vi "SCM Host Calibration.vi"() -> ()   [LabVIEW 2015]
uses:
  <vilib>/addons/Software Calibration Management/XControls/TBL2D.xctl
  <vilib>/addons/Software Calibration Management/XControls/TBL1D.xctl
panel:
  in  "stop":bool
  in  "Calibration":T1(tab)
  in  "SCalibrationFileName":string
  in  "bResetLapStatistics":bool
  in  "bResetNLap":bool
  in  "bResetFastestLap":bool
  in  "tLapReference":u32
  in  "CExtraNotes":string
  in  "CSessionDescription":string
  in  "CDriverName":string
  in  "CCircuit":string
  in  "CCarName":string
  in  "kPID_D":sgl
  in  "kPID_I":sgl
  in  "kPID_P":sgl
  in  "PLimitCalculatedCurrent":sgl
  in  "PLimit":sgl
  in  "bPowerLimiterDisable":bool
  out "rTPS2":sgl(slide) scale=0.0..1.0
  out "rTPS1":sgl(slide) scale=0.0..1.0
  in  "rTPS2Min":sgl
  in  "rTPS2Max":sgl
  out "rTPS2Unscaled":sgl
  in  "rTPS1Min":sgl
  in  "rTPS1Max":sgl
  out "rTPS1Unscaled":sgl
  in  "NDashRateDividerRotaryMap":cluster{"X":sgl[], "Y":sgl[]}(xcontrol)
  in  "NThrottleMapRotaryMap":cluster{"X":sgl[], "Y":sgl[]}(xcontrol)
  in  "NTorqueMapRotaryMap":cluster{"X":sgl[], "Y":sgl[]}(xcontrol)
  in  "Torque Maps":enum32{"0", "1", "2", "3", "4", "5"}(tab)
  in  "rTorqueMap0":cluster{"X":sgl[], "Y":sgl[], "Z":sgl[][]}(xcontrol)
  in  "rTorqueMap1":cluster{"X":sgl[], "Y":sgl[], "Z":sgl[][]}(xcontrol)
  in  "rTorqueMap2":cluster{"X":sgl[], "Y":sgl[], "Z":sgl[][]}(xcontrol)
  in  "rTorqueMap3":cluster{"X":sgl[], "Y":sgl[], "Z":sgl[][]}(xcontrol)
  in  "rTorqueMap4":cluster{"X":sgl[], "Y":sgl[], "Z":sgl[][]}(xcontrol)
  in  "rTorqueMap5":cluster{"X":sgl[], "Y":sgl[], "Z":sgl[][]}(xcontrol)
  in  "rThrottleMap5":cluster{"X":sgl[], "Y":sgl[]}(xcontrol)
  in  "rThrottleMap4":cluster{"X":sgl[], "Y":sgl[]}(xcontrol)
  in  "rThrottleMap3":cluster{"X":sgl[], "Y":sgl[]}(xcontrol)
  in  "rThrottleMap2":cluster{"X":sgl[], "Y":sgl[]}(xcontrol)
  in  "rThrottleMap1":cluster{"X":sgl[], "Y":sgl[]}(xcontrol)
  in  "rThrottleMap0":cluster{"X":sgl[], "Y":sgl[]}(xcontrol)
  in  "xTireDiameter":sgl
  in  "VSteerWheelMiddle":sgl
  in  "tLapMin":u32
  in  "VSupplyOffset":sgl
  in  "bWheelFRFail":bool
  in  "bWheelFLFail":bool
  in  "VPrechargeMinimum":sgl
  in  "bMCVoltageCheckDisable":bool
  in  "TCellMaxFanThreshold":sgl
  in  "pBrakeRBrakeLightThresh":sgl
  in  "pBrakeFBrakeLightThresh":sgl
  in  "gAccelThreshold":sgl
  in  "pBrakeFBrakeBalThresh":sgl
  in  "tLapTriggerOverride":u32
  in  "tTDMSTelemetryPeriod":u32
  in  "tMCTelemetryPeriod":u32
  in  "tFPGATelemetryPeriod":u32
  in  "tRTDS":u32
  in  "tPrecharge":u32
  in  "pBrakeFActivation":sgl
  in  "NMCCANOffset":u32
  in  "bDCDCEnable":bool
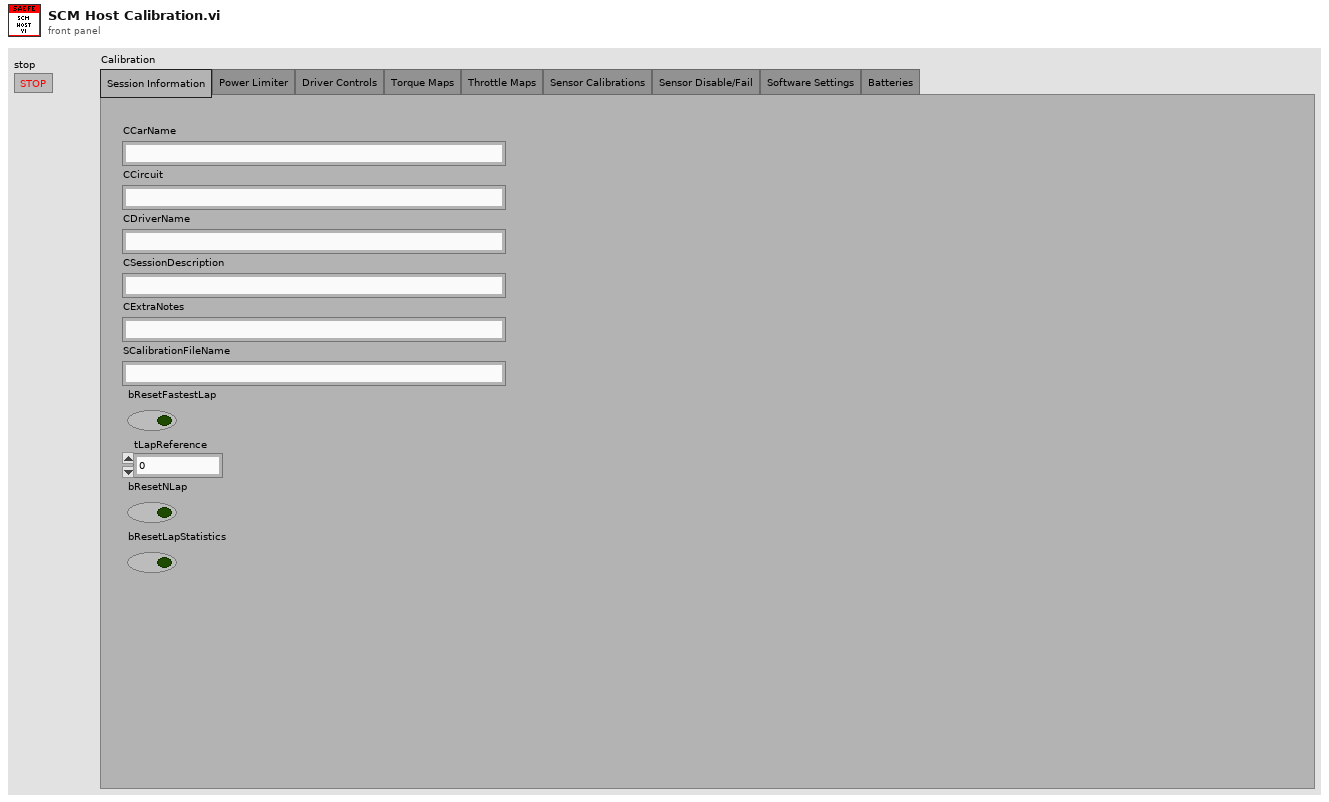
[diagram p1: front panel]
types:
  T1 = enum32{"Session Information", "Power Limiter", "Driver Controls", "Torque Maps", "Throttle Maps", "Sensor Calibrations", "Sensor Disable/Fail", "Software Settings", "Batteries"}
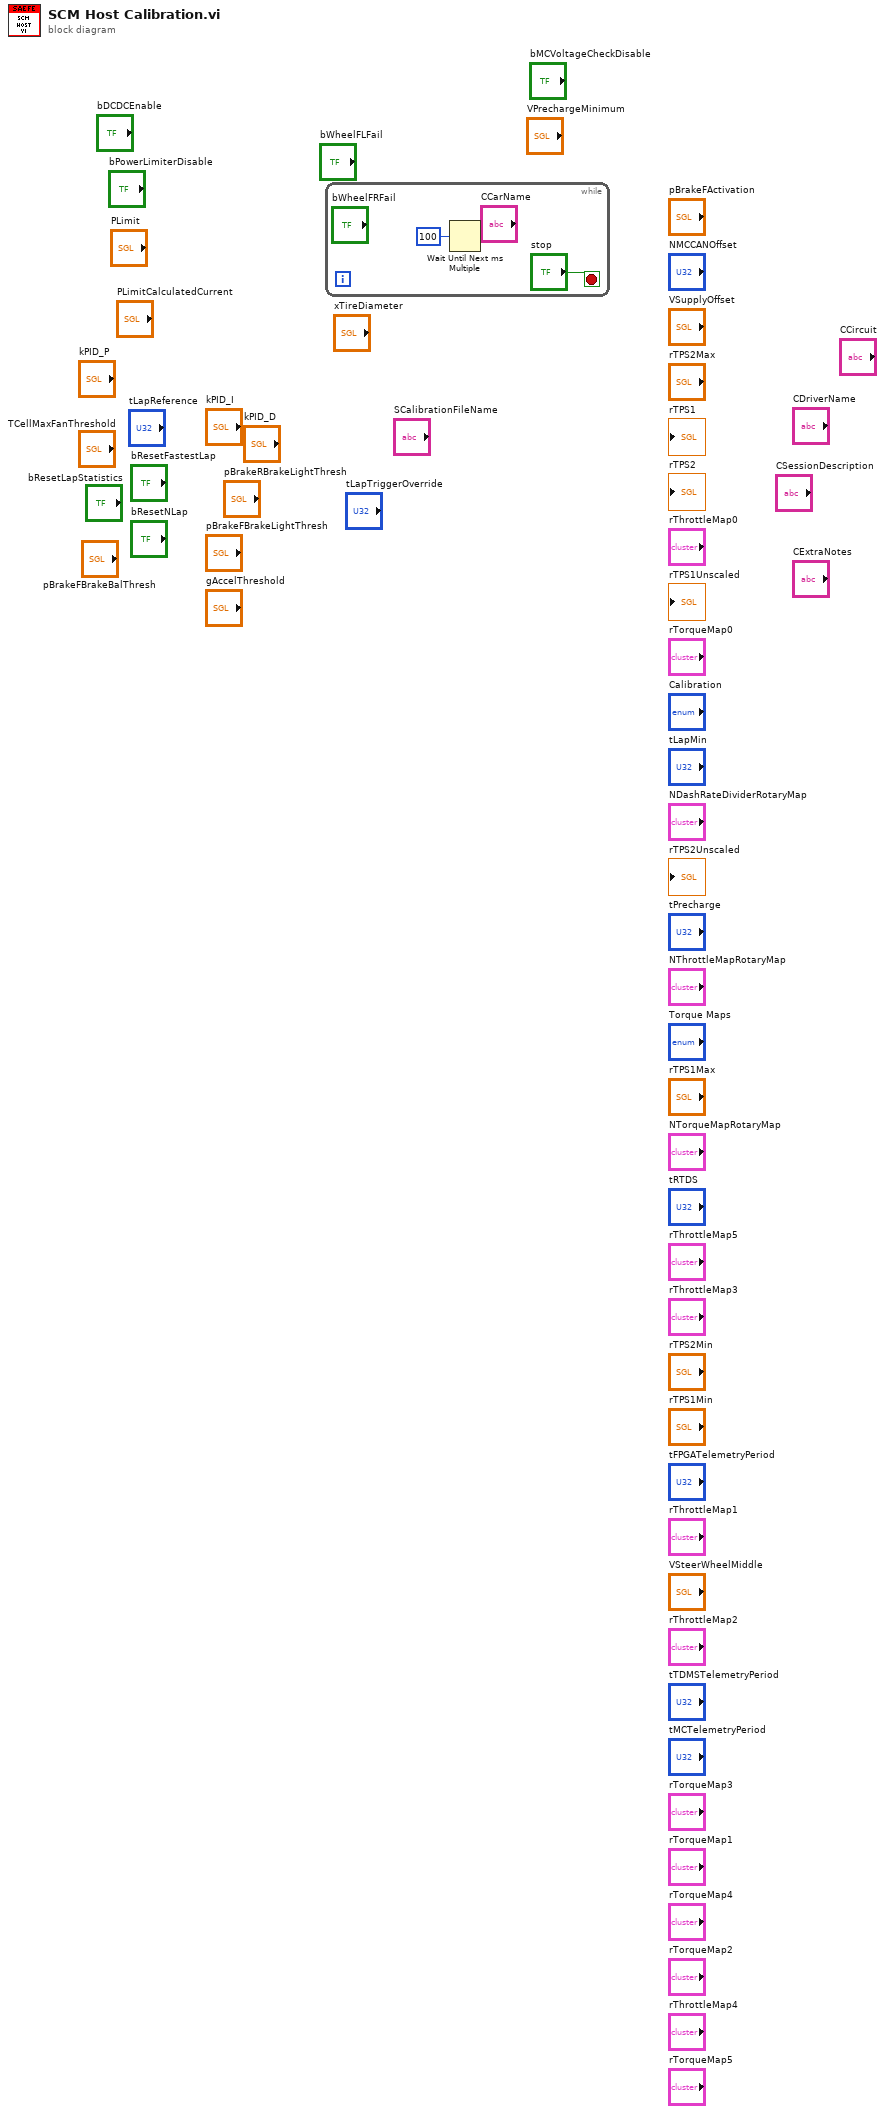
[diagram p0: block diagram]
diagram:
  n1 = while {
    stop <- "stop" stop-if-true
    n2 = Wait Until Next ms Multiple(millisecond multiple=u32 100) -> ()  [unwired: 1 out]
  }
